vi "Set Tag Symbol.vi"(8 "error in (no error)":errorcluster, 10 "Symbol Index":i32, 11 "Tag_LVOOP in":refnum<class "Tree Tag Class.lvclass">) -> (0 "error out":errorcluster, 3 "Tag_LVOOP out":refnum<class "Tree Tag Class.lvclass">)   [LabVIEW 2012, in "Tree Tools.lvlib" / "Tree Tag Class.lvclass"]
uses:
  Tree Tag Class.lvclass
  Tree Tag Class.lvclass/Tree Tag Class.ctl
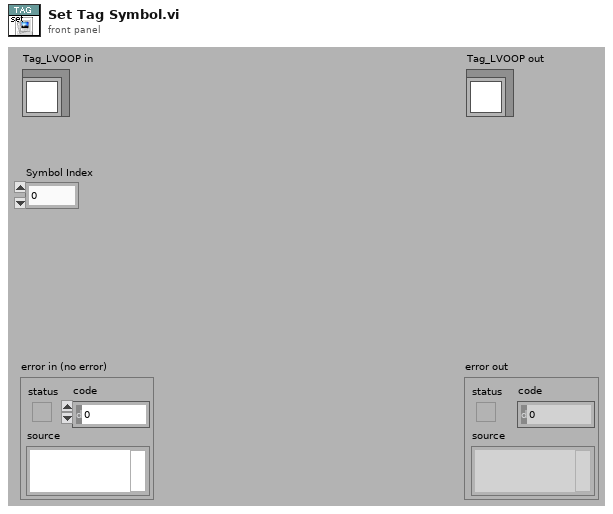
[diagram p1: front panel]
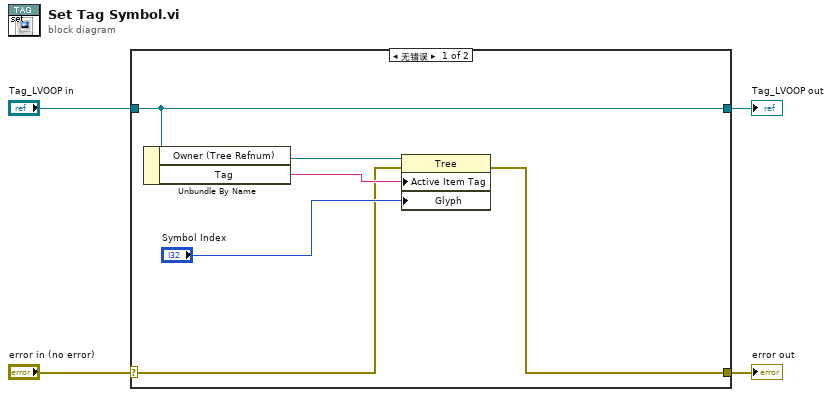
[diagram p0: block diagram]
diagram:
  n1 = case shown="无错误" "error in (no error)" {
    selector: "error in (no error)" -> [w6 w12]
    tunnel: [w5 w12] -> w3
    tunnel: [w10 w11] -> w1
    tunnel: "Tag_LVOOP in" -> [w10 w11]
    frame No Error {
      n2 = Unbundle By Name(w10) -> ("Owner (Tree Refnum)"=w9:refnum<vi>, "Tag"=w8:string)
      n3 = property class="Tree"(reference=w9, error in=w6, "Active Item Tag"=w8, "Glyph"="Symbol Index") -> (error out=w5:errorcluster)  [unwired: 1 out]
    }
    frame Error {
    }
  }
  "error out" <- w3
  "Tag_LVOOP out" <- w1
